vi "正玄函数强度强度图vi.vi"() -> ()   [LabVIEW 2023]
panel:
  out "Intensity Graph":dbl[][](graph)
  out "Intensity Chart":dbl[][](graph)
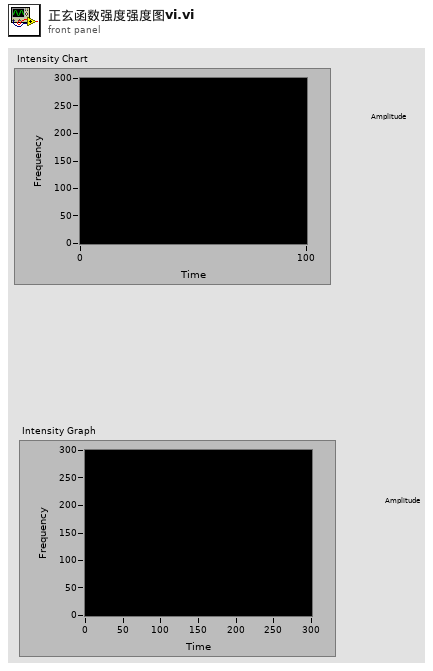
[diagram p1: front panel]
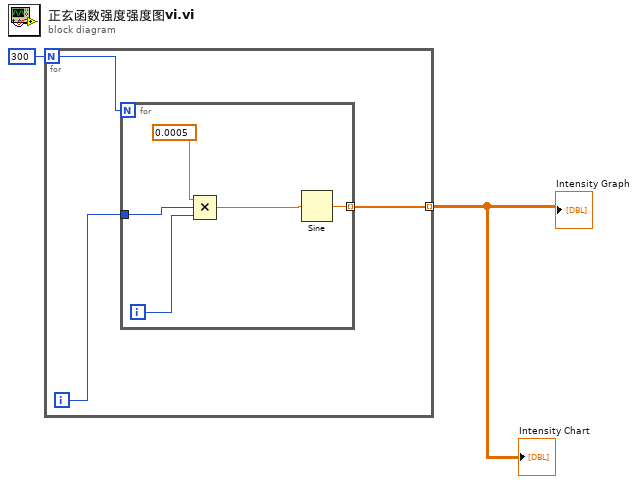
[diagram p0: block diagram]
diagram:
  n1 = for {
    N: 300 -> [w5]
    tunnel: [w3] -> w1 mode=indexing
    i -> [w4]
    n2 = for {
      N: w5 -> [_]
      tunnel: [w9] -> w3 mode=indexing
      tunnel: w4 -> [w7]
      i -> [w8]
      n3 = Compound Arithmetic op=MULTIPLY(0.0005, w7, w8) -> (w10:dbl)
      n4 = Sine(x=w10) -> (sin(x)=w9:dbl)
    }
  }
  "Intensity Graph" <- w1
  "Intensity Chart" <- w1
